vi "PH_BeamlineInformation.get Head Index by Voltage Service Name.vi"(0 "i ref in":refnum<vi>, 2 "Voltage Service Name":string, 5 "error in (no error)":errorcluster) -> (13 "Voltage linked?":bool, 14 "i ref out":refnum<vi>, 16 "index of element":i32, 17 "GUI Ref":refnum<vi>, 18 "Voltage [V]":dbl, 19 "error out":errorcluster)   [LabVIEW 2014, in "PH_BeamlineInformation.lvlib"]
uses:
  PH_BeamlineInformation.lvlib
  PH_PP_Common/PH_PP_Common.PSU Tags.ctl
  PH_PP_Common/PH_PP_Common.lvlib
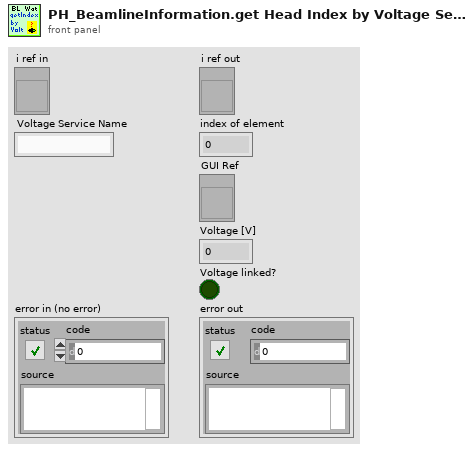
[diagram p1: front panel]
types:
  T1 = typedef "PH_PP_Common.lvlib/PH_PP_Common.PSU Tags.ctl" = enum16{"voltage-indicator", "peak-detect", "current", "voltage", "inihibit-indicator", "end-of-charge", "HV-on-indicator", "overtemperature", "interlock-indicator", "load-fault", "sum-fault", "HV-off-indicator", "DC-ok", "inhibit", "HV-on", "interlock", "reset", "Status", "Limits"}
  T2 = typedef "PH_BeamlineInformation.lvlib/PH_BeamlineInformation.i attribute.ctl" = cluster{"BL GUI Elements of Services":cluster{"Service Name":string, "GUI Elements":refnum<vi>[], "Status":i32}[], "Powermeters":T3, "Efficiency":T4, "Heads":T5[]}
  T3 = typedef "PH_BeamlineInformation.lvlib/PH_BeamlineInformation.Powermeter.ctl" = cluster{"ns FE":cluster{"GUI Ref":refnum<vi>, "Value":dbl}, "fs FE":cluster{"GUI Ref":refnum<vi>, "Value":dbl}, "PA":cluster{"GUI Ref":refnum<vi>, "Value":dbl}, "MA":cluster{"GUI Ref":refnum<vi>, "Value":dbl}, "Z6 green":cluster{"GUI Ref":refnum<vi>, "Value":dbl}, "Z6 IR":cluster{"GUI Ref":refnum<vi>, "Value":dbl}, "Z6 COS":cluster{"GUI Ref":refnum<vi>, "Value":dbl}}
  T4 = typedef "PH_BeamlineInformation.lvlib/PH_BeamlineInformation.Efficiency.ctl" = cluster{"PA Gain":cluster{"GUI Ref":refnum<vi>, "Value":dbl}, "MA Gain":cluster{"GUI Ref":refnum<vi>, "Value":dbl}, "Z6 green Conversion":cluster{"GUI Ref":refnum<vi>, "Value":dbl}, "Z6 Comp Losses":cluster{"GUI Ref":refnum<vi>, "Value":dbl}}
  T5 = typedef "PH_BeamlineInformation.lvlib/PH_BeamlineInformation.Head.ctl" = cluster{"PowerUnit":T6, "in use":cluster{"Value":bool, "GUI Ref":refnum<vi>, "linked":bool}, "voltage":cluster{"Value":dbl, "GUI Ref":refnum<vi>, "linked":bool}}
  T6 = typedef "PH_PP_Common.lvlib/PH_PP_Common.PUs.ctl" = enum16{"no Info", "PA-19mm-1", "PA-19mm-2", "PA-45mm-PILC", "PA-45mm-MAIN", "MA-PU-1", "MA-PU-2", "MA-PU-3", "MA-PU-4", "MA-PU-5", "MA-PU-6", "MA-FR", "MA-PILC", "PA-45mm-DP"}
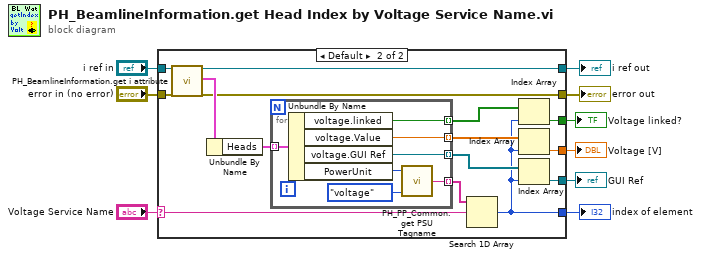
[diagram p0: block diagram]
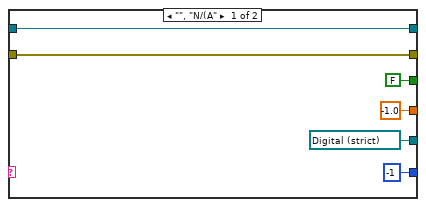
[diagram p2: hidden frame]
diagram:
  n1 = case shown="Default" "Voltage Service Name" {
    selector: "Voltage Service Name" -> [_ w25]
    tunnel: [w15 w28] -> w9
    tunnel: "i ref in" -> [w15 w27]
    tunnel: [-1 ("index of element") w17] -> w7
    tunnel: "error in (no error)" -> [w14 w26]
    tunnel: [w14 w21] -> w5
    tunnel: [refnum<vi> refnum ("GUI Ref") w23] -> w3
    tunnel: [-1.0 ("Value") w20] -> w2
    tunnel: [FALSE ("linked") w16] -> w1
    frame "", "N/(A" {
    }
    frame Default {
      n2 = call "PH_BeamlineInformation.get i attribute.vi"("i ref in"=w27, "error in (no error)"=w26) -> ("i ref out"=w28:refnum<vi>, "i attribute"=w29:T2, "error out"=w21:errorcluster)  [unwired: 15 in]
      n3 = Unbundle By Name(w29) -> ("Heads"=w19:T5[])
      n4 = for {
        tunnel: w19 -> [w37] mode=indexing
        tunnel: [w33] -> w30 mode=indexing
        tunnel: [w36] -> w24 mode=indexing
        tunnel: [w35] -> w22 mode=indexing
        tunnel: [w31] -> w18 mode=indexing
        n5 = Unbundle By Name(w37) -> ("voltage.linked"=w31:bool, "voltage.Value"=w35:dbl, "voltage.GUI Ref"=w36:refnum<vi>, "PowerUnit"=w34:T6)
        n6 = call "PH_PP_Common.get PSU Tagname.vi"("PSU Tag"=PH_PP_Common.PSU_Tags."voltage", "PU"=w34) -> ("PSU Tagname"=w33:string)  [unwired: 1 in]
      }
      n7 = Search 1D Array(1D array=w30, element=w25) -> (index of element=w17:i32)  [unwired: 1 in]
      n8 = Index Array(array=w18, index=w17) -> (element=w16:bool)
      n9 = Index Array(array=w22, index=w17) -> (element=w20:dbl)
      n10 = Index Array(array=w24, index=w17) -> (element=w23:refnum<vi>)
    }
  }
  "i ref out" <- w9
  "error out" <- w5
  "index of element" <- w7
  "GUI Ref" <- w3
  "Voltage [V]" <- w2
  "Voltage linked?" <- w1
